vi "Deqeue message.vi"(8 "error in (no error)":errorcluster, 11 "RxTx in":refnum<class "RxTx.lvclass">) -> (0 "error out":errorcluster, 3 "RxTx out":refnum<class "RxTx.lvclass">)   [LabVIEW 2018, in "RxTx.lvclass"]
doc: "Este VI retira o último elemento de uma fila."
uses:
  RxTx.lvclass
  RxTx.lvclass/RxTx.ctl
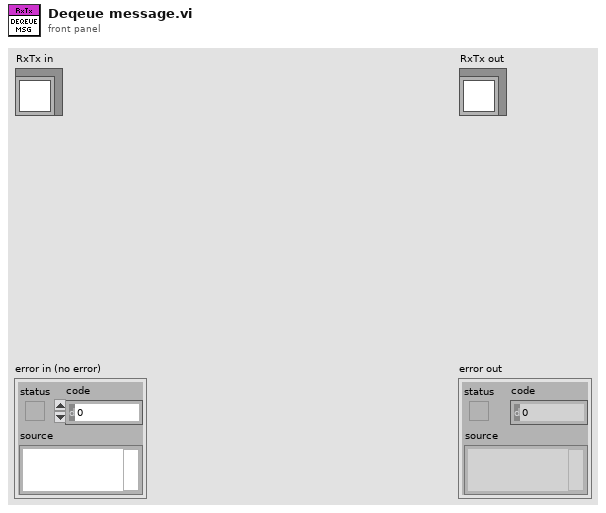
[diagram p1: front panel]
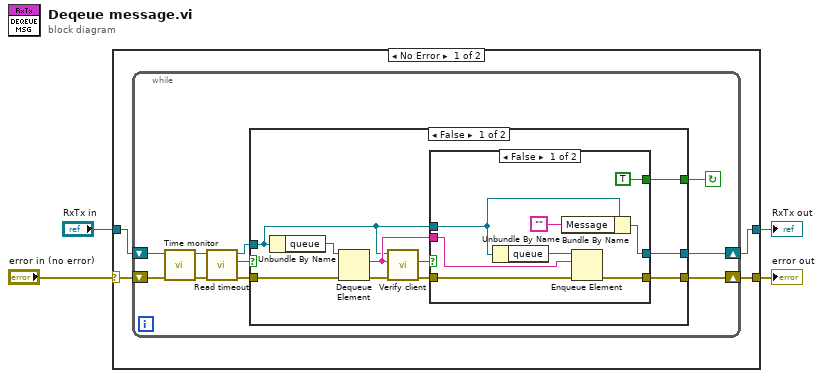
[diagram p0: block diagram]
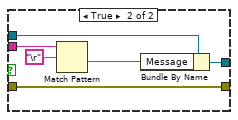
[diagram p2: hidden frame]
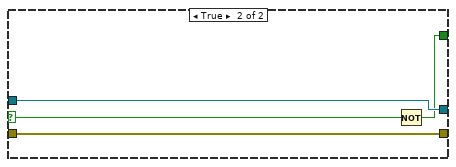
[diagram p3: hidden frame]
diagram:
  n1 = case shown="No Error" "error in (no error)" {
    selector: "error in (no error)" -> [w8 w48]
    tunnel: [w5 w48] -> w3
    tunnel: [w7 w47] -> w1
    tunnel: "RxTx in" -> [w6 w47]
    frame No Error {
      n2 = while {
        shift-right: [w11] -> w7
        shift-left: w6 -> [w17]
        shift-right: [w10] -> w5
        shift-left: w8 -> [w18]
        stop <- w9 continue-if-true
        n3 = call "Time monitor.vi"("error in (no error)"=w18, "RxTx in"=w17) -> ("error out"=w16:errorcluster, "RxTx out"=w15:refnum<class "RxTx.lvclass">)  [unwired: 8 in]
        n4 = call "Read timeout.vi"("error in (no error)"=w16, "RxTx in"=w15) -> ("error out"=w13:errorcluster, "timeout ?"=w12:bool, "RxTx out"=w14:refnum<class "RxTx.lvclass">)  [unwired: 7 in]
        n5 = case shown="False" w12 {
          selector: w12 -> [_ w43]
          tunnel: w14 -> [w23 w46]
          tunnel: w13 -> [w22 w45]
          tunnel: [w21 w44] -> w9
          tunnel: [w20 w46] -> w11
          tunnel: [w19 w45] -> w10
          frame False {
            n6 = Unbundle By Name(w23) -> ("queue"=w28:refnum<queue>)
            n7 = Dequeue Element(queue=w28, error in (no error)=w22) -> (element=w25:string, error out=w27:errorcluster)  [unwired: 1 in, 2 out]
            n8 = call "Verify client.vi"("error in (no error)"=w27, "Message"=w25, "RxTx in"=w23) -> ("error out"=w24:errorcluster, "verify receiver"=w26:bool)  [unwired: 6 in, 1 out]
            n9 = case shown="False" w26 {
              tunnel: w25 -> [w34 w39]
              tunnel: [w31 w42] -> w20
              tunnel: w23 -> [w33 w41]
              tunnel: w24 -> [w36 w40]
              tunnel: [w30 w40] -> w19
              tunnel: [TRUE _] -> w21
              frame False {
                n10 = Unbundle By Name(w33) -> ("queue"=w35:refnum<queue>)
                n11 = Bundle By Name(cluster=w33, "Message"="") -> (w31:refnum<class "RxTx.lvclass">)
                n12 = Enqueue Element(queue=w35, element=w34, error in (no error)=w36) -> (error out=w30:errorcluster)  [unwired: 1 in, 2 out]
              }
              frame True {
                n13 = Match Pattern(string=w39, regular expression="\r") -> (after substring=w37:string)  [unwired: 1 in, 3 out]
                n14 = Bundle By Name(cluster=w41, "Message"=w37) -> (w42:refnum<class "RxTx.lvclass">)
              }
            }
          }
          frame True {
            n15 = Not(x=w43) -> (.not. x?=w44:bool)
          }
        }
      }
    }
    frame Error {
    }
  }
  "error out" <- w3
  "RxTx out" <- w1
